vi "Start Cyclic Data Query.vi"(8 "error in (no error)":errorcluster, 10 "Query Period (ms)":i32=1000, 11 "Modbus in":refnum<class "Modbus.lvclass">) -> (0 "error out":errorcluster, 3 "Modbus out":refnum<class "Modbus.lvclass">)   [LabVIEW 2020, in "Modbus.lvlib" / "Modbus.lvclass"]
uses:
  Modbus.lvclass
  Sensor/Sensor/Sensor.lvclass
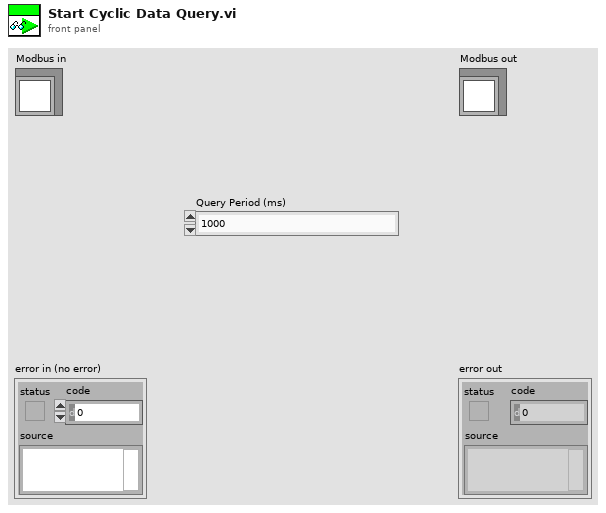
[diagram p1: front panel]
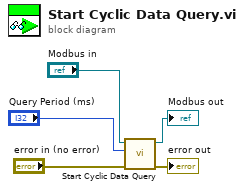
[diagram p0: block diagram]
diagram:
  n1 = call-parent "Start Cyclic Data Query.vi"("error in (no error)"="error in (no error)", "Query Period (ms)"="Query Period (ms)", "Sensor in"="Modbus in") -> ("error out"=→"error out":errorcluster, "Sensor out"=→"Modbus out":refnum<class "Modbus.lvclass">)  [unwired: 7 in]
